vi "histogram_gestos_prawd(SubVI).vi"(9 "rozdzielczosc":dbl, 10 "samples":i32, 11 "Gaussian noise pattern":dbl[](array[numeric])) -> (1 "dystrybuanta":cluster{dbl[], dbl[]}(graph), 2 "gestosc prawd":cluster{dbl[], dbl[]}(graph), 3 "histogram":cluster{dbl[], i32[]}(graph))   [LabVIEW 2025]
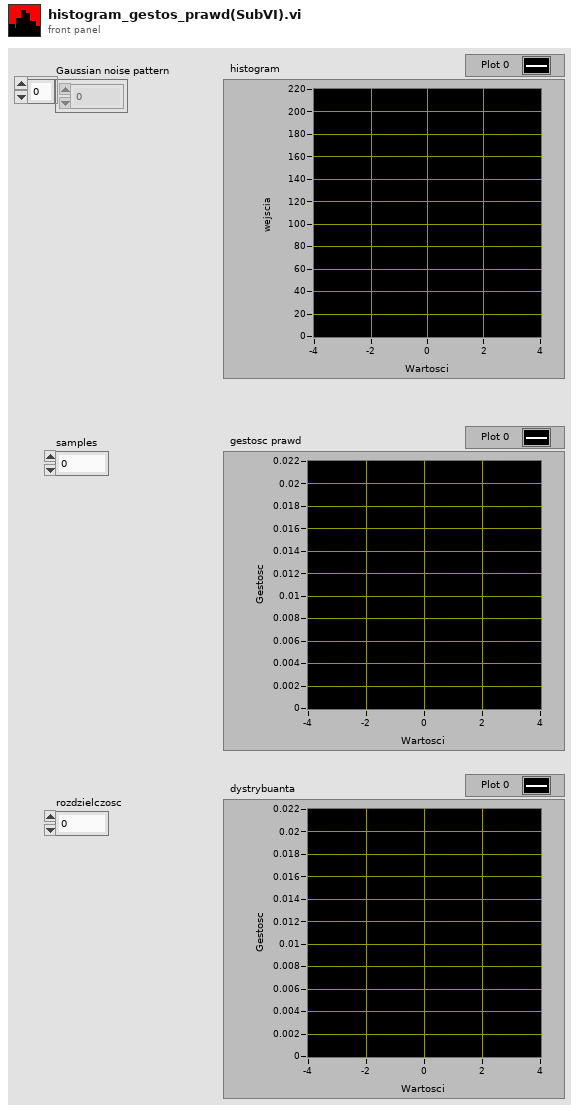
[diagram p1: front panel]
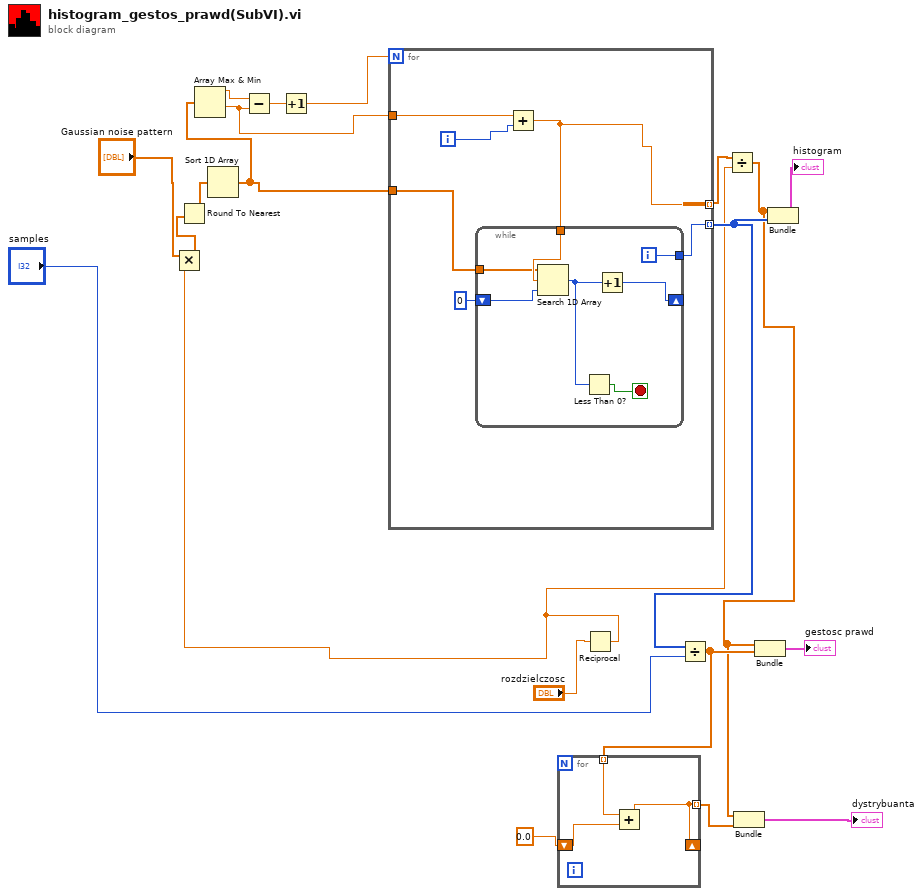
[diagram p0: block diagram]
diagram:
  n1 = Reciprocal(x="rozdzielczosc") -> (1/x=w17:dbl)
  n2 = Multiply(x="Gaussian noise pattern", y=w17) -> (x*y=w14:dbl[])
  n3 = Round To Nearest(number=w14) -> (nearest integer value=w15:dbl[])
  n4 = Sort 1D Array(array=w15) -> (sorted array=w11:dbl[])
  n5 = Array Max & Min(array=w11) -> (max value=w9:dbl, min value=w10:dbl)  [unwired: 2 out]
  n6 = Subtract(x=w9, y=w10) -> (x-y=w7:dbl)
  n7 = Increment(x=w7) -> (x+1=w8:dbl)
  n8 = for {
    N: w8 -> [_]
    tunnel: w10 -> [w26]
    tunnel: w11 -> [w25]
    tunnel: [w24] -> w20 mode=indexing
    tunnel: [w23] -> w13 mode=indexing
    i -> [w21]
    n9 = Add(x=w26, y=w21) -> (x+y=w23:dbl)
    n10 = while {
      tunnel: w23 -> [w32]
      tunnel: w25 -> [w31]
      shift-right: [w29] -> _
      shift-left: 0 -> [w30]
      tunnel: [w27] -> w24
      i -> [w27]
      stop <- w33 stop-if-true
      n11 = Search 1D Array(1D array=w31, element=w32, start index (0)=w30) -> (index of element=w28:i32)
      n12 = Less Than 0?(x=w28) -> (x < 0?=w33:bool)
      n13 = Increment(x=w28) -> (x+1=w29:i32)
    }
  }
  n14 = Divide(x=w20, y="samples") -> (x/y=w4:dbl[])
  n15 = for {
    shift-right: [w34] -> _
    shift-left: 0.0 -> [w36]
    tunnel: w4 -> [w35] mode=indexing
    tunnel: [w34] -> w1 mode=indexing
    n16 = Add(x=w35, y=w36) -> (x+y=w34:dbl)
  }
  n17 = Divide(x=w13, y=w17) -> (x/y=w3:dbl[])
  n18 = Bundle(w3, w1) -> (→"dystrybuanta":cluster{dbl[], dbl[]})  [unwired: 1 in]
  n19 = Bundle(w3, w4) -> (→"gestosc prawd":cluster{dbl[], dbl[]})  [unwired: 1 in]
  n20 = Bundle(w3, w20) -> (→"histogram":cluster{dbl[], i32[]})  [unwired: 1 in]
